vi "FVI_read_distance.vi"(11 "refnum name":string) -> (3 "Numeric":dbl)   [LabVIEW 2018]
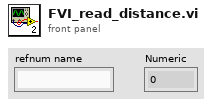
[diagram p1: front panel]
types:
  T1 = typedef "WPI_AnalogChannelDevRef.ctl" = cluster{"DevStatus":errorcluster, "Analog Channel":T2}
  T2 = typedef "FPGA_AIChannel.ctl" = enum8{"AI 0", "AI 1", "AI 2", "AI 3", "AI MXP 0", "AI MXP 1", "AI MXP 2", "AI MXP 3", "Invalid"}
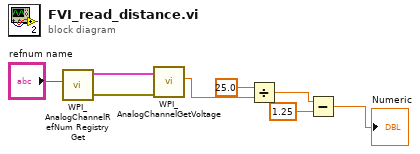
[diagram p0: block diagram]
diagram:
  n1 = call <vilib>:"WPI_AnalogChannelRefNum Registry Get.vi"("refnum name"="refnum name") -> ("error out"=w2:errorcluster, "AIDeviceRef"=w1:T1)  [unwired: 9 in]
  n2 = call <vilib>:"WPI_AnalogChannelGetVoltage.vi"("error in (no error)"=w2, "AIDeviceRef"=w1) -> ("Voltage"=w4:dbl)  [unwired: 7 in, 2 out]
  n3 = Divide(x=25.0, y=w4) -> (x/y=w7:dbl)
  n4 = Subtract(x=w7, y=1.25) -> (x-y=→"Numeric":dbl)
